vi "VI Tree - xxx- Files__ogtk.vi"   [LabVIEW 2016]
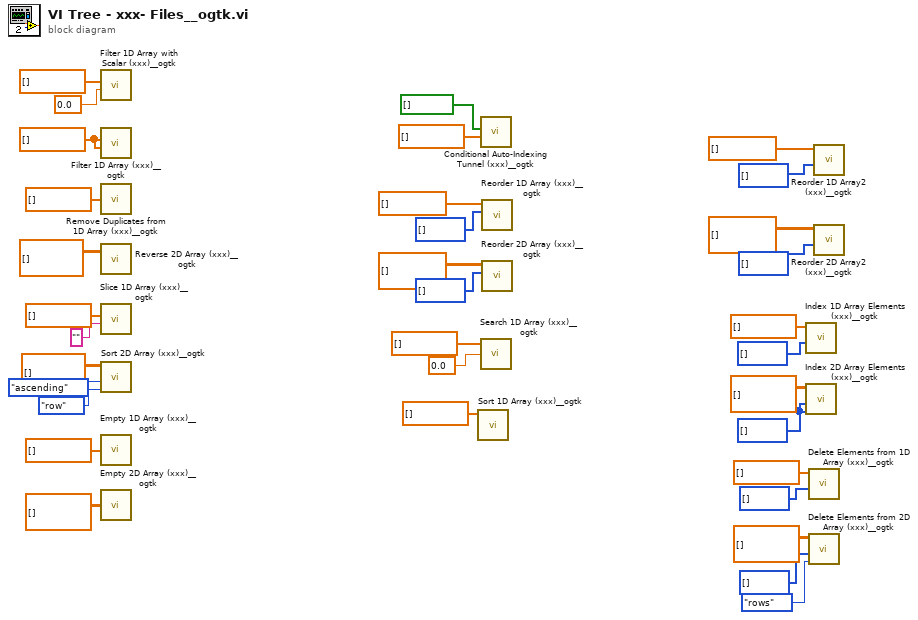
[diagram p0: block diagram]
diagram:
  w1 = i32[] [] ("indices")
  w33 = dbl[] [] ("Array")
  n1 = call <userlib>:"Filter 1D Array with Scalar (xxx)__ogtk.vi"("items to filter"=0.0 ("Numeric"), "array"=dbl[] [] ("Array")) -> ()  [unwired: 4 in, 2 out]
  n2 = call <userlib>:"Filter 1D Array (xxx)__ogtk.vi"("items to filter"=w33, "array"=w33) -> ()  [unwired: 4 in, 2 out]
  n3 = call <userlib>:"Remove Duplicates from 1D Array (xxx)__ogtk.vi"("Input Array"=dbl[] []) -> ()  [unwired: 2 out]
  n4 = call <userlib>:"Reverse 2D Array (xxx)__ogtk.vi"("Array"=dbl[][] []) -> ()  [unwired: 2 in, 1 out]
  n5 = call <userlib>:"Slice 1D Array (xxx)__ogtk.vi"("slice"="", "array"=dbl[] []) -> ()  [unwired: 5 in, 1 out]
  n6 = call <userlib>:"Sort 2D Array (xxx)__ogtk.vi"("Sort By in"=enum16{"row", "column"}."row", "Order"=enum16{"ascending", "descending"}."ascending", "Array in"=dbl[][] []) -> ()  [unwired: 5 in, 4 out]
  n7 = call <userlib>:"Empty 1D Array (xxx)__ogtk.vi"("Array"=dbl[] []) -> ()  [unwired: 8 in, 1 out]
  n8 = call <userlib>:"Empty 2D Array (xxx)__ogtk.vi"("Array"=dbl[][] []) -> ()  [unwired: 8 in, 1 out]
  n9 = call <userlib>:"Sort 1D Array (xxx)__ogtk.vi"("Array in"=dbl[] []) -> ()  [unwired: 9 in, 2 out]
  n10 = call <userlib>:"Conditional Auto-Indexing Tunnel (xxx)__ogtk.vi"("Array in"=dbl[] [], "Elements to keep"=bool[] []) -> ()  [unwired: 5 in, 1 out]
  n11 = call <userlib>:"Search 1D Array (xxx)__ogtk.vi"("Array"=dbl[] [], "Element Data"=0.0) -> ()  [unwired: 7 in, 1 out]
  n12 = call <userlib>:"Reorder 1D Array (xxx)__ogtk.vi"("Sorted Pointers in"=i32[] [], "Array in"=dbl[] []) -> ()  [unwired: 8 in, 2 out]
  n13 = call <userlib>:"Reorder 2D Array (xxx)__ogtk.vi"("Sorted Pointers in"=i32[] [], "Array in"=dbl[][] []) -> ()  [unwired: 7 in, 3 out]
  n14 = call <userlib>:"Index 1D Array Elements (xxx)__ogtk.vi"("indices"=i32[] [], "array"=dbl[] []) -> ()  [unwired: 9 in, 1 out]
  n15 = call <userlib>:"Index 2D Array Elements (xxx)__ogtk.vi"("indices 1"=w1, "indices 0"=w1, "array"=dbl[][] []) -> ()  [unwired: 8 in, 1 out]
  n16 = call <userlib>:"Delete Elements from 1D Array (xxx)__ogtk.vi"("indices"=i32[] [], "array"=dbl[] []) -> ()  [unwired: 8 in, 2 out]
  n17 = call <userlib>:"Delete Elements from 2D Array (xxx)__ogtk.vi"("delete (rows or columns)"=enum16{"rows", "columns"}."rows", "indices"=i32[] [], "array"=dbl[][] []) -> ()  [unwired: 7 in, 2 out]
  n18 = call <userlib>:"Reorder 1D Array2 (xxx)__ogtk.vi"("indices"=i32[] [] ("Sorted Pointers in"), "array"=dbl[] [] ("Array in")) -> ()  [unwired: 9 in, 1 out]
  n19 = call <userlib>:"Reorder 2D Array2 (xxx)__ogtk.vi"("indices"=i32[] [] ("Sorted Pointers in"), "array"=dbl[][] [] ("Array in")) -> ()  [unwired: 9 in, 1 out]
